vi "Reactivity Fitting.vi"() -> ()   [LabVIEW 2020]
uses:
  <vilib>/Utility/miscctls.llb/LVAnnotationListTypeDef.ctl
  global/SettingVariable.vi
  <vilib>/Analysis/NI_AALPro.lvlib
panel:
  out "反应性相对偏差":dbl[](array[numeric]) caption="相对偏差 (%)"
  out "最小二乘周期":dbl[](array[numeric]) caption="最小二乘法拟合 (s)"
  out "广义指数周期":dbl[](array[numeric]) caption="广义指数拟合 (s)"
  out "实测平均反应性":dbl[](array[numeric]) caption="实测平均值 (pcm)"
  out "周期法反应性":dbl[](array[numeric]) caption="周期法 (pcm)"
  out "采样间隔":dbl
  out "开始时间":timestamp
  in  "打开文件":bool
  out "历史波形图":cluster{dbl, dbl, dbl[][]}(graph)
  out "左选标时刻":timestamp caption="左选标时刻：" format="%<%.2X %x>T"
  out "数据点数":i32 caption="选中的数据点数："
  out "反应性记录表":string[][](table) caption="计算结果记录表"
  in  "保存表格":bool
  in  "添加记录":bool
  out "提示信息":string="打开文件后，拖动波形图中的游标选取临界段、动态段和终端段数据进行计算。"
  out "文件信息":string
  # "周期计算结果"
  # "反应性计算结果"
  # "坐标轴与图例"
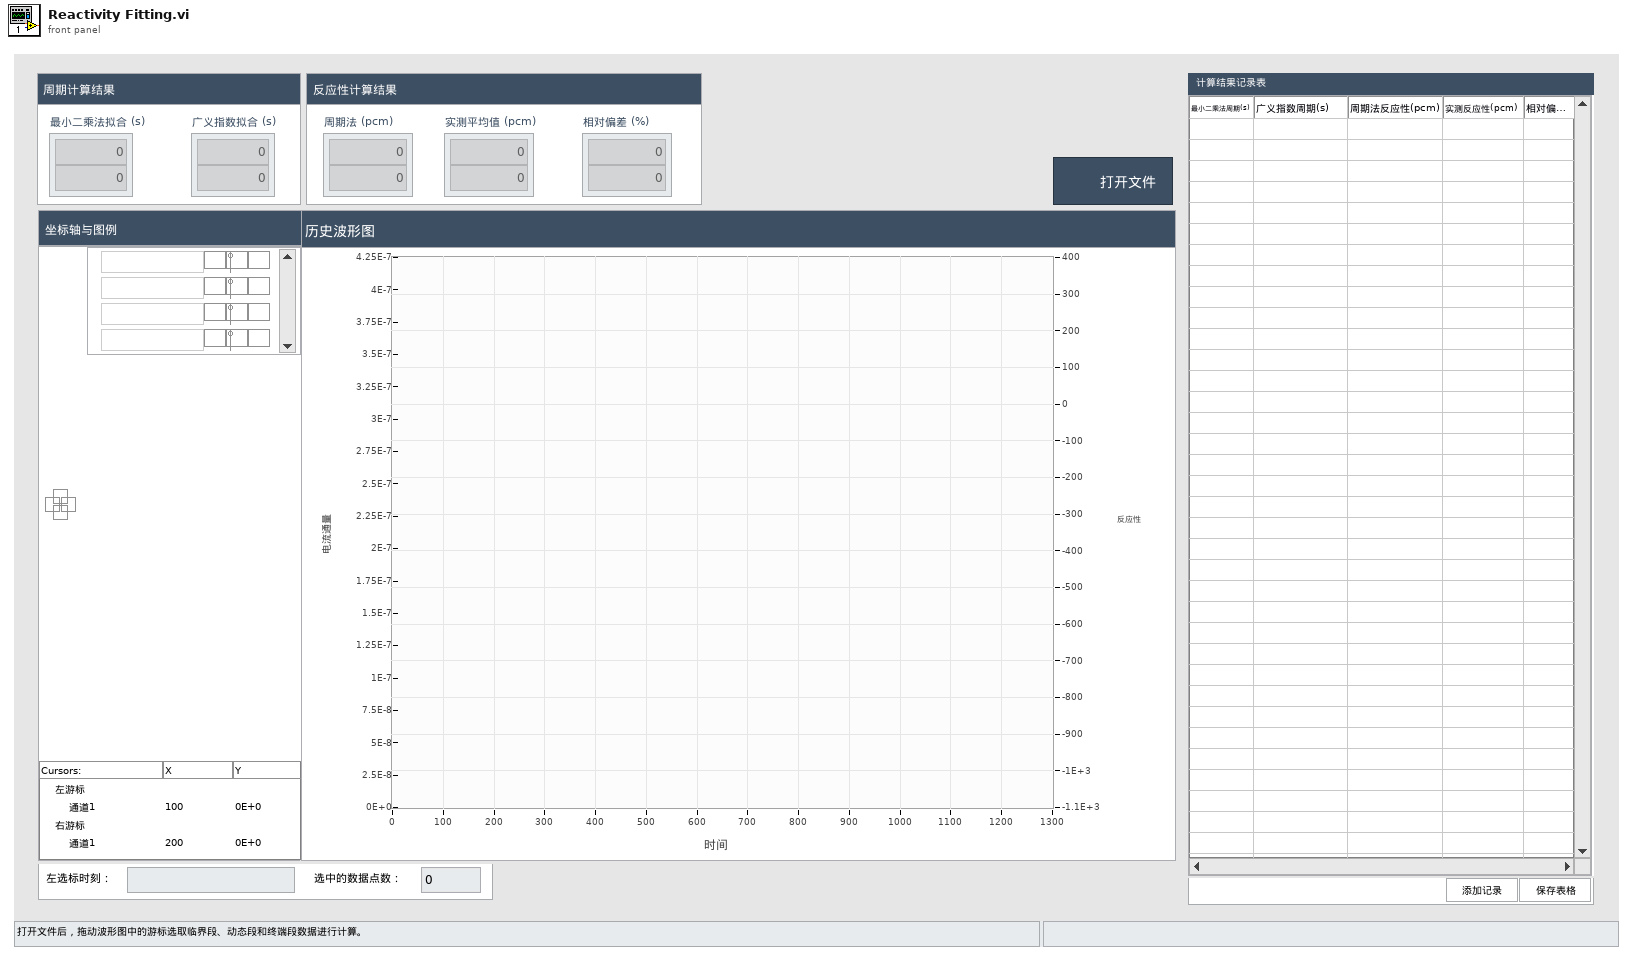
[diagram p1: front panel]
types:
  T1 = typedef "LVAnnotationListTypeDef.ctl" = cluster{"Name":string, "Color":u32, "Style":u8, "Point Style":u8, "Name Visible":bool, "Allow Drag":bool, "Annotation Mode":u32, "Plot":i32, "Index":i32, "Position":cluster{"X":dbl, "Y":dbl}, "X Scale":u32, "Y Scale":u32, "Show Arrow":bool, "Lock Name":bool, "Plot Area":i32, "Label Offset":cluster{"X":dbl, "Y":dbl}}[]
  T2 = cluster{"Name":string, "Color":u32, "Style":u8, "Point Style":u8, "Name Visible":bool, "Allow Drag":bool, "Annotation Mode":u32, "Plot":i32, "Index":i32, "Position":cluster{"X":dbl, "Y":dbl}, "X Scale":u32, "Y Scale":u32, "Show Arrow":bool, "Lock Name":bool, "Plot Area":i32, "Label Offset":cluster{"X":dbl, "Y":dbl}}
  T3 = cluster{"amp min":dbl, "amp max":dbl, "damping min":dbl, "damping max":dbl, "offset min":dbl, "offset max":dbl}
  T4 = enum16{"open", "replace", "create", "open or create", "replace or create", "replace or create with confirmation"}
  T5 = typedef "LVCursorListTypeDef.ctl" = cluster{"Name":string, "Color":u32, "Style":u8, "Point Style":u8, "Name Visible":bool, "Allow Drag":bool, "Cursor Mode":u32, "Plot":i32, "Index":i32, "Position":cluster{"X":dbl, "Y":dbl}, "X Scale":u32, "Y Scale":u32, "Watch Plots":i32[], "Watch All Plots":bool, "Plot Area":i32, "Label Offset":cluster{"X":dbl, "Y":dbl}}[]
  T6 = cluster{"Name":string, "Color":u32, "Style":u8, "Point Style":u8, "Name Visible":bool, "Allow Drag":bool, "Cursor Mode":u32, "Plot":i32, "Index":i32, "Position":cluster{"X":dbl, "Y":dbl}, "X Scale":u32, "Y Scale":u32, "Watch Plots":i32[], "Watch All Plots":bool, "Plot Area":i32, "Label Offset":cluster{"X":dbl, "Y":dbl}}
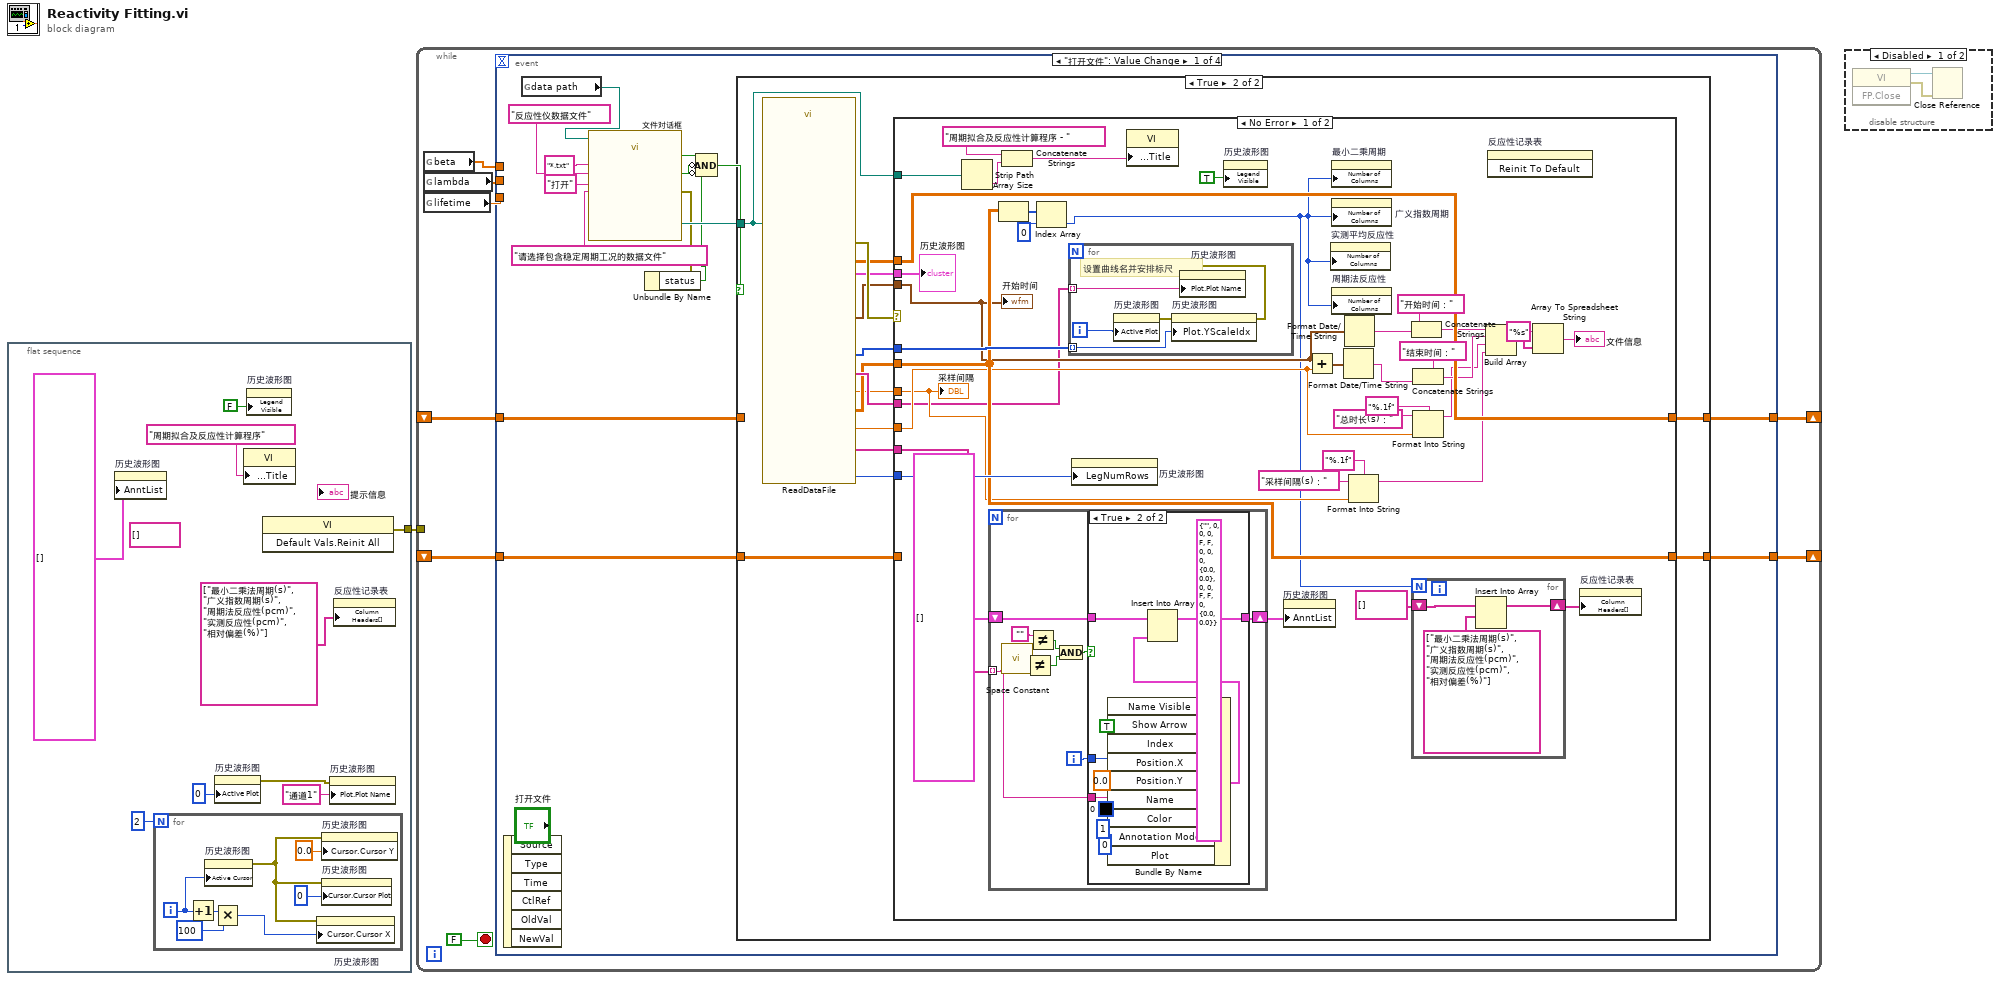
[diagram p0: block diagram]
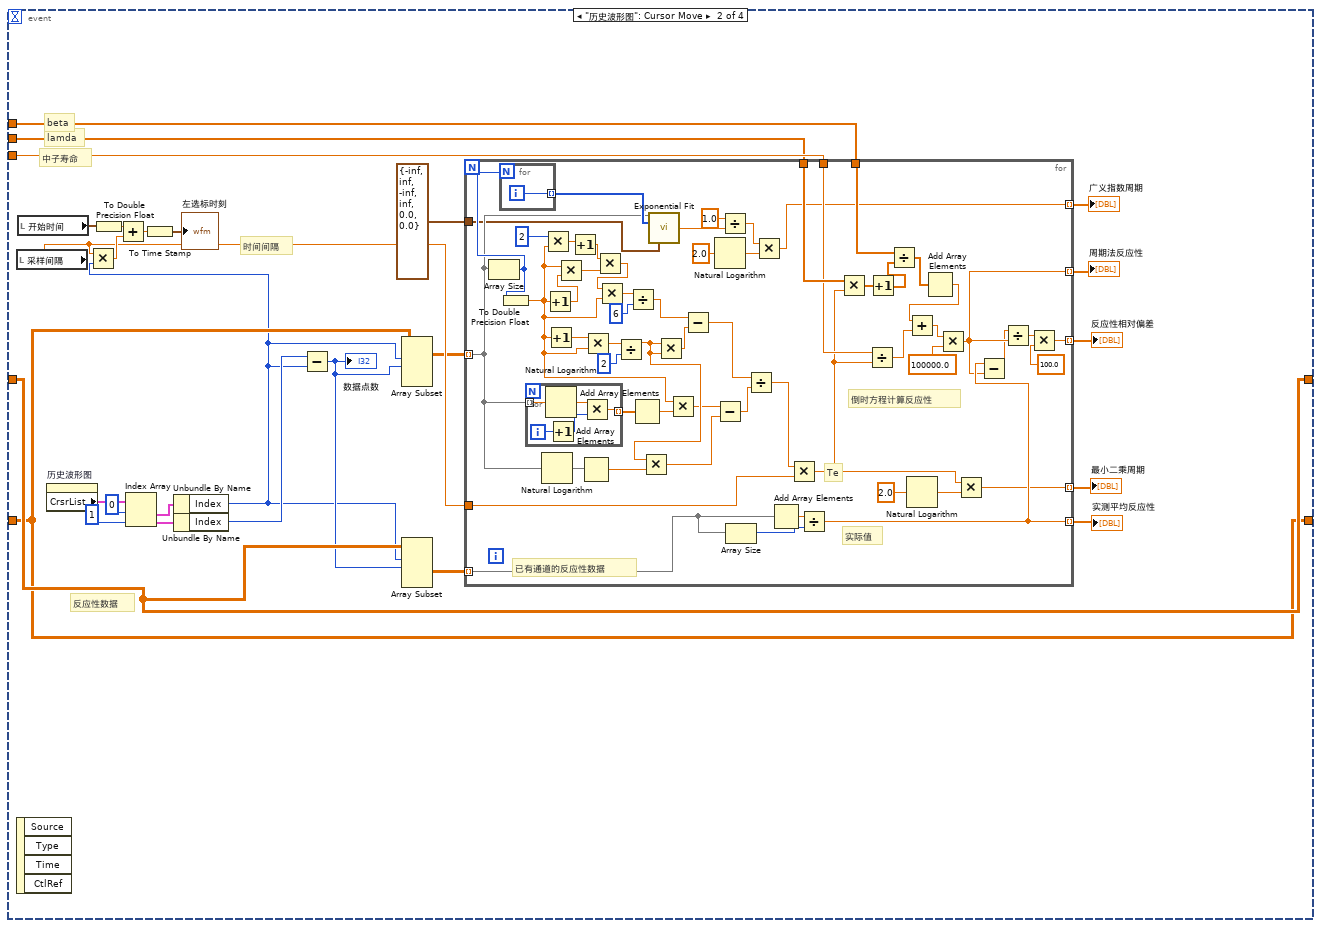
[diagram p5: hidden frame]
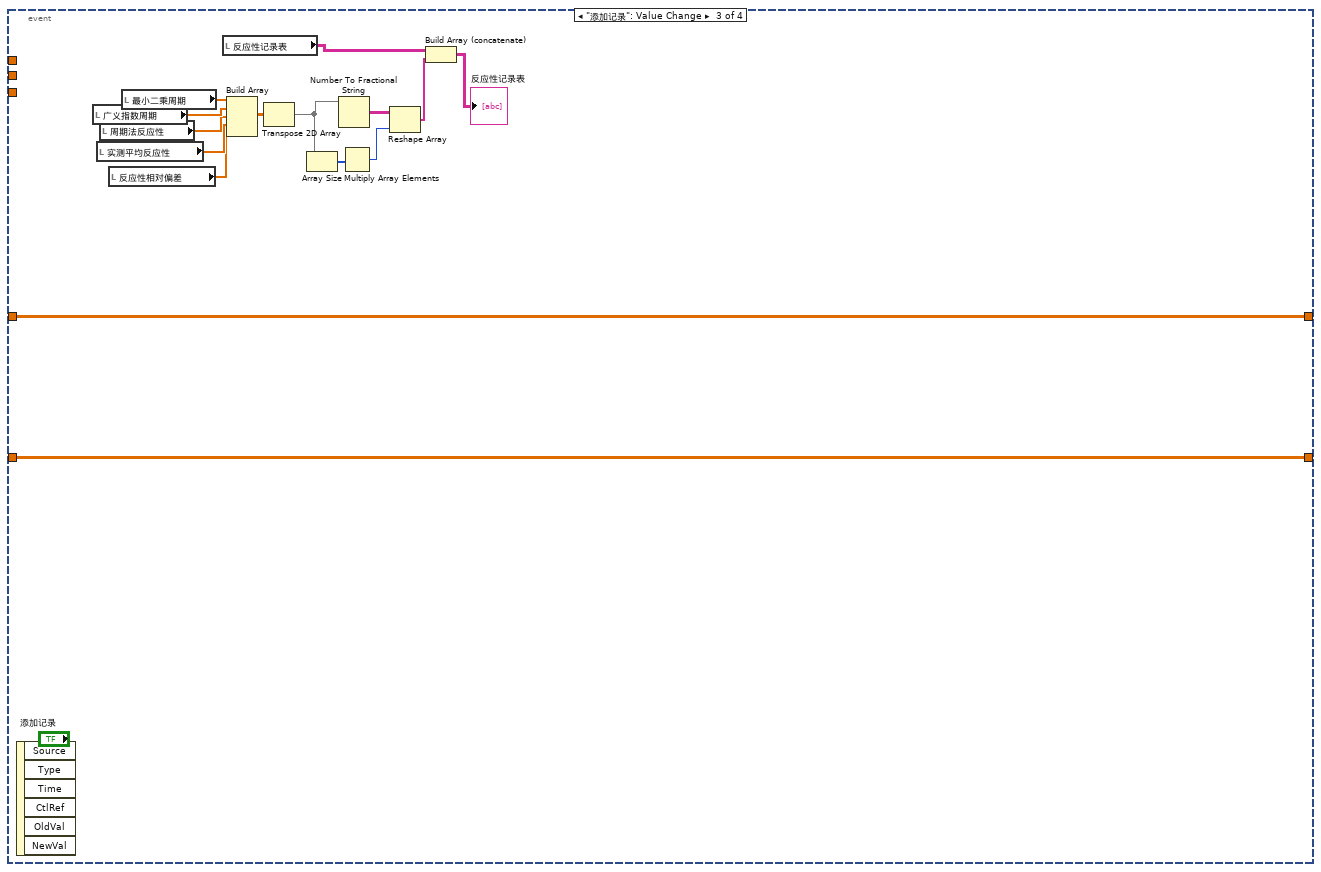
[diagram p6: hidden frame]
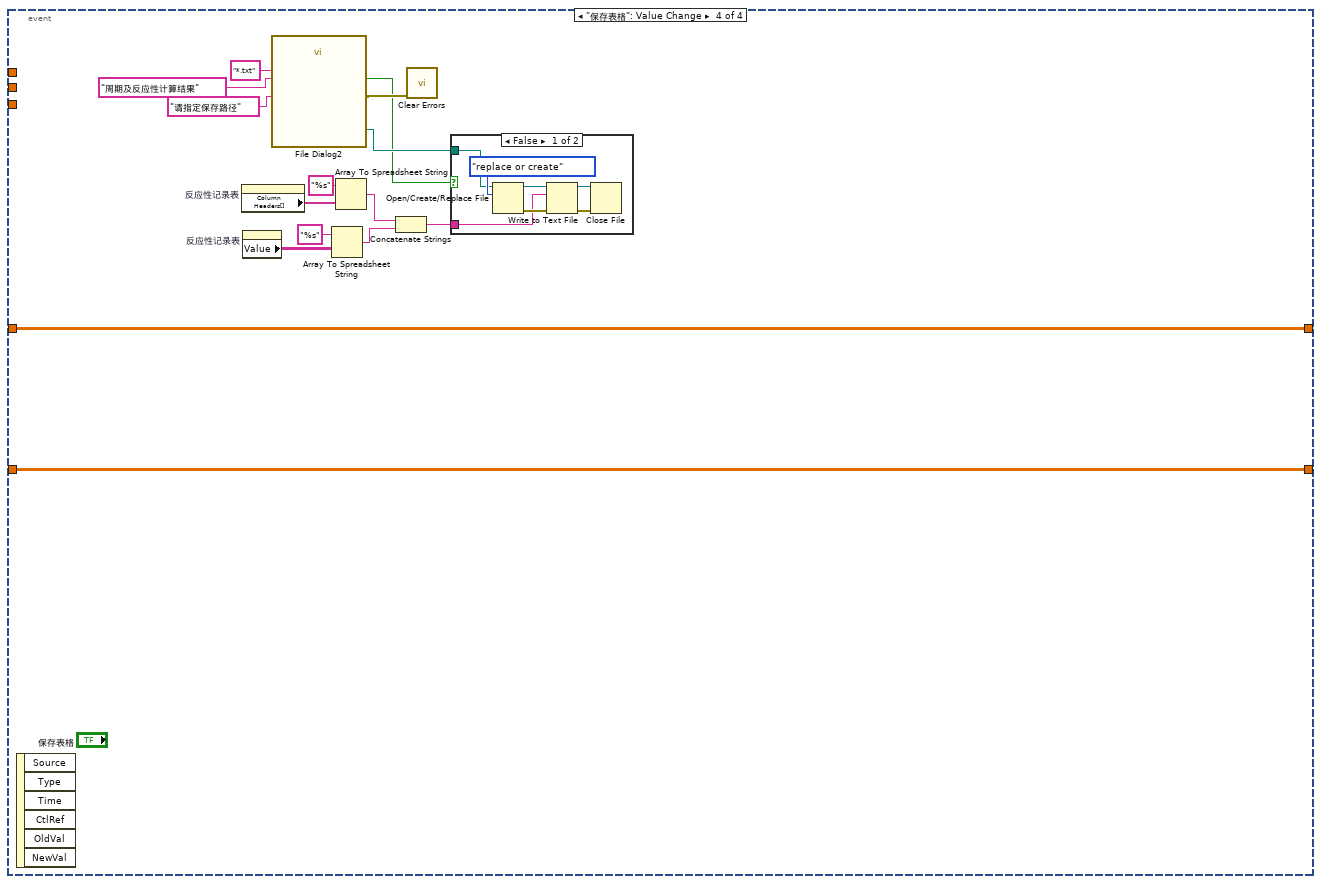
[diagram p7: hidden frame]
diagram:
  n1 = flat-sequence {
    tunnel: [w6] -> w1
    frame #0 {
      (unwired) string[] [] ("Strings []")
      n2 = property on="历史波形图" class="WFGraph (strict)"("AnntList"=T1 [] ("Annotation List")) -> ()  [unwired: 2 in, 2 out]
      n3 = for {
        N: 2 -> [_]
        i -> [w15]
        n4 = Increment(x=w15) -> (x+1=w14:i32)
        n5 = property on="历史波形图" class="WFGraph (strict)"("Active Cursor"=w15) -> (error out=w11:errorcluster)  [unwired: 2 in, 1 out]
        n6 = Multiply(x=w14, y=100) -> (x*y=w12:i32)
        n7 = property on="历史波形图" class="WFGraph (strict)"(error in=w11, "Cursor.Cursor X"=w12) -> ()  [unwired: 1 in, 2 out]
        n8 = property on="历史波形图" class="WFGraph (strict)"(error in=w11, "Cursor.Cursor Y"=0.0 ("Cursor.Cursor Position:Cursor Y")) -> ()  [unwired: 1 in, 2 out]
        n9 = property on="历史波形图" class="WFGraph (strict)"(error in=w11, "Cursor.Cursor Plot"=0 ("Cursor.Cursor Index")) -> ()  [unwired: 1 in, 2 out]
      }
      n10 = property on="历史波形图" class="WFGraph (strict)"("Active Plot"=u32 0) -> (error out=w8:errorcluster)  [unwired: 2 in, 1 out]
      n11 = property class="VI"("Front Panel.Title"="周期拟合及反应性计算程序" ("Front Panel Window:Title")) -> ()  [unwired: 2 in, 2 out]
      n12 = property on="历史波形图" class="WFGraph (strict)"("Legend Visible"=FALSE ("Legend:Visible")) -> ()  [unwired: 2 in, 2 out]
      n13 = invoke class="VI" method="Default Vals.Reinit All"() -> (error out=w6:errorcluster)  [unwired: 3 in, 2 out]
      n14 = property on="历史波形图" class="WFGraph (strict)"(error in=w8, "Plot.Plot Name"="通道1") -> ()  [unwired: 1 in, 2 out]
      n15 = property on="反应性记录表" class="Tbl (strict)"("Column Headers[]"=string[] ["最小二乘法周期(s)", "广义指数周期(s)", "周期法反应性(pcm)", "实测反应性(pcm)", "相对偏差(%)"] ("行首字符串[]")) -> ()  [unwired: 2 in, 2 out]
    }
  }
  n16 = while {
    shift-right: [w24] -> _
    shift-left: _ -> [w23]
    shift-right: [w22] -> _
    shift-left: _ -> [w21]
    tunnel: w1 -> [_]
    stop <- FALSE stop-if-true
    n17 = global read "SettingVariable.vi" "beta"() -> (w20:dbl[])
    n18 = global read "SettingVariable.vi" "lambda"() -> (w19:dbl[])
    n19 = global read "SettingVariable.vi" "lifetime"() -> (w18:dbl)
    n20 = event shown="[0] \"打开文件\": Value Change" {
      selector: _ -> [_ _ _ _]
      dyn-events: _ -> [_ _ _ _]
      timeout: _ -> [_ _ _ _]
      tunnel: [w35 w129 w231 w246] -> w24
      tunnel: w23 -> [w34 w129 w231 w246]
      tunnel: [w33 w143 w232 w247] -> w22
      tunnel: w21 -> [w32 w143 w232 w247]
      tunnel: w20 -> [_ w134 _ _]
      tunnel: w18 -> [_ w135 _ _]
      tunnel: w19 -> [_ w133 _ _]
      event "打开文件": Value Change {
        n21 = event-data() -> ()  [unwired: 1 in, 6 out]
        n22 = global read "SettingVariable.vi" "data path"() -> (w26:path)
        n23 = call "文件对话框"("start path"=w26, "prompt"="请选择包含稳定周期工况的数据文件", "button label"="打开", "pattern (all files)"="*.txt", "pattern label"="反应性仪数据文件") -> ("selected path"=w40:path, "exists"=w30:bool, "cancelled"=w29:bool, "error out"=w31:errorcluster)  [unwired: 7 in]
        n24 = Unbundle By Name(w31) -> ("status"=w28:bool)
        n25 = Compound Arithmetic op=AND(w30, invert w29, invert w28) -> (w27:bool)
        n26 = case shown="True" w27 {
          tunnel: w40 -> [_ w43]
          tunnel: [w42 w49] -> w35
          tunnel: w34 -> [w42 w48]
          tunnel: [w41 w45] -> w33
          tunnel: w32 -> [w41 _]
          frame False {
          }
          frame True {
            n27 = call "ReadDataFile.vi"("file path (dialog if empty)"=w43) -> ("曲线对应标尺编号"=w52:i32[], "曲线名"=w51:string[], "通量数据"=w50:dbl[][], "时间间隔"=w47:dbl, "曲线数"=w54:i32, "开始时间"=w44:timestamp, "反应性数据"=w46:dbl[][], "总时长(s)"=w55:dbl, "error out"=w57:errorcluster, "备注数组"=w53:string[], "波形簇"=w56:cluster{dbl, dbl, dbl[][]})  [unwired: 2 in, 2 out]
            n28 = case shown="No Error" w57 {
              tunnel: w56 -> [w95 _]
              tunnel: w55 -> [w77 _]
              tunnel: w54 -> [w94 _]
              tunnel: w53 -> [w91 _]
              tunnel: w52 -> [w90 _]
              tunnel: w51 -> [w64 _]
              tunnel: w50 -> [w87 _]
              tunnel: [w87 w126] -> w49
              tunnel: w48 -> [_ w126]
              tunnel: w47 -> [w75 _]
              tunnel: w46 -> [w86 w125]
              tunnel: [w86 w125] -> w45
              tunnel: w44 -> [w82 _]
              tunnel: w43 -> [w59 _]
              frame No Error {
                n29 = Strip Path(path=w59) -> (name=w60:string)  [unwired: 1 out]
                n30 = for {
                  tunnel: w91 -> [w107] mode=indexing
                  shift-right: [w109] -> w93
                  shift-left: T1 [] ("注释列表") -> [w110]
                  i -> [w111]
                  n31 = call <vilib>:"Space Constant.vi"() -> ("String"=w112:string)
                  n32 = Not Equal?(x=w112, y=w107) -> (x != y?=w105:bool)
                  n33 = Not Equal?(x="", y=w107) -> (x != y?=w106:bool)
                  n34 = And(x=w106, y=w105) -> (x .and. y?=w104:bool)
                  n35 = case shown="True" w104 {
                    tunnel: w107 -> [_ w119]
                    tunnel: w111 -> [_ w121]
                    tunnel: w110 -> [w113 w124]
                    tunnel: [w113 w123] -> w109
                    frame False {
                    }
                    frame True {
                      w122 = TRUE ("Show Arrow")
                      n36 = Bundle By Name(cluster=T2 {"Name"="", "Color"=0, "Style"=0, "Point Style"=0, "Name Visible"=FALSE, "Allow Drag"=FALSE, "Annotation Mode"=0, "Plot"=0, "Index"=0, "Position"={"X"=0.0, "Y"=0.0}, "X Scale"=0, "Y Scale"=0, "Show Arrow"=FALSE, "Lock Name"=FALSE, "Plot Area"=0, "Label Offset"={"X"=0.0, "Y"=0.0}} ("元素"), "Name Visible"=w122, "Show Arrow"=w122, "Index"=w121, "Position.X"=w121, "Position.Y"=0.0 ("Y"), "Name"=w119, "Color"=u32 0, "Annotation Mode"=u32 1, "Plot"=0) -> (w120:T2)
                      n37 = Insert Into Array(array=w124, new element=w120) -> (w123:T1)  [unwired: 1 in]
                    }
                  }
                }
                n38 = Array Size(array=w87) -> (size(s)=w89:i32[])
                n39 = Concatenate Strings("周期拟合及反应性计算程序 - " ("string"), w60) -> (w61:string)
                n40 = Index Array(array=w89, index=0 ("索引")) -> (element=w63:i32)
                n41 = for {
                  tunnel: w90 -> [w101] mode=indexing
                  tunnel: w64 -> [w99] mode=indexing
                  i -> [w100]
                  # "设置曲线名并安排标尺"
                  n42 = property on="历史波形图" class="WFGraph (strict)"("Active Plot"=w100) -> (error out=w103:errorcluster)  [unwired: 2 in, 1 out]
                  n43 = property on="历史波形图" class="WFGraph (strict)"(error in=w103, "Plot.YScaleIdx"=w101) -> (error out=w102:errorcluster)  [unwired: 1 in, 1 out]
                  n44 = property on="历史波形图" class="WFGraph (strict)"(error in=w102, "Plot.Plot Name"=w99) -> ()  [unwired: 1 in, 2 out]
                }
                n45 = property on="历史波形图" class="WFGraph (strict)"("LegNumRows"=w94) -> ()  [unwired: 2 in, 2 out]
                n46 = property class="VI"("Front Panel.Title"=w61) -> ()  [unwired: 2 in, 2 out]
                n47 = property on="历史波形图" class="WFGraph (strict)"("Legend Visible"=TRUE ("Legend:Visible")) -> ()  [unwired: 2 in, 2 out]
                n48 = property on="历史波形图" class="WFGraph (strict)"("AnntList"=w93) -> ()  [unwired: 2 in, 2 out]
                n49 = Add(x=w82, y=w77) -> (x+y=w83:timestamp)
                n50 = property on="实测平均反应性" class="Arr (strict)"("Number of Columns"=w63) -> ()  [unwired: 2 in, 2 out]
                n51 = property on="最小二乘周期" class="Arr (strict)"("Number of Columns"=w63) -> ()  [unwired: 2 in, 2 out]
                n52 = property on="广义指数周期" class="Arr (strict)"("Number of Columns"=w63) -> ()  [unwired: 2 in, 2 out]
                n53 = property on="周期法反应性" class="Arr (strict)"("Number of Columns"=w63) -> ()  [unwired: 2 in, 2 out]
                n54 = Format Date/Time String(seconds (now)=w83) -> (date/time string=w78:string)  [unwired: 2 in]
                n55 = Format Date/Time String(seconds (now)=w82) -> (date/time string=w80:string)  [unwired: 2 in]
                n56 = Format Into String(format string="%.1f", initial string="采样间隔(s)：", w75) -> (resulting string=w68:string)  [unwired: 1 in, 1 out]
                n57 = Concatenate Strings("开始时间：" ("string"), w80) -> (w73:string)
                n58 = for {
                  N: w63 -> [_]
                  shift-right: [w96] -> w84
                  shift-left: string[] [] ("行首字符串[]") -> [w97]
                  n59 = Insert Into Array(array=w97, new element=string[] ["最小二乘法周期(s)", "广义指数周期(s)", "周期法反应性(pcm)", "实测反应性(pcm)", "相对偏差(%)"] ("行首字符串[]")) -> (w96:string[])  [unwired: 1 in]
                }
                n60 = Concatenate Strings("结束时间：" ("string"), w78) -> (w70:string)
                n61 = Format Into String(format string="%.1f", initial string="总时长(s)：", w77) -> (resulting string=w69:string)  [unwired: 1 in, 1 out]
                n62 = Build Array(w73, w70, w69, w68) -> (w72:string[])
                n63 = invoke on="反应性记录表" class="Tbl (strict)" method="Reinit To Default"() -> ()  [unwired: 3 in, 3 out]
                n64 = Array To Spreadsheet String(array=w72, 3:"%s" ("format string")) -> (spreadsheet string=→"文件信息":string)  [unwired: 1 in]
                n65 = property on="反应性记录表" class="Tbl (strict)"("Column Headers[]"=w84) -> ()  [unwired: 2 in, 2 out]
                "历史波形图" <- w95
                "开始时间" <- w82
                "采样间隔" <- w75
              }
              frame Error {
              }
            }
          }
        }
      }
      event "历史波形图": Cursor Move {
        # "lamda"
        # "beta"
        # "中子寿命"
        # "反应性数据"
        # "时间间隔"
        n66 = local read "采样间隔"() -> (w132:dbl)
        n67 = event-data() -> ()  [unwired: 1 in, 4 out]
        n68 = local read "开始时间"() -> (w142:timestamp)
        n69 = property on="历史波形图" class="WFGraph (strict)"() -> ("CrsrList"=w149:T5)  [unwired: 2 in, 2 out]
        n70 = To Double Precision Float(number=w142) -> (double precision float=w148:dbl)
        n71 = Index Array(array=w149, index #1=0 ("index"), index #2=1 ("index")) -> (element #1=w151:T6, element #2=w153:T6)
        n72 = Unbundle By Name(w151) -> ("Index"=w127:i32)
        n73 = Multiply(x=w132, y=w127) -> (x*y=w145:dbl)
        n74 = Add(x=w148, y=w145) -> (x+y=w147:dbl)
        n75 = To Time Stamp(1:w147) -> (0:→"左选标时刻":timestamp)
        n76 = Unbundle By Name(w153) -> ("Index"=w144:i32)
        n77 = Subtract(x=w144, y=w127) -> (x-y=w128:i32)
        "数据点数" <- w128
        n78 = Array Subset(array=w129, index (row)=w127, length (row)=w128) -> (w130:dbl[][])  [unwired: 2 in]
        n79 = Array Subset(array=w143, index (row)=w127, length (row)=w128) -> (w131:dbl[][])  [unwired: 2 in]
        n80 = for {
          tunnel: w130 -> [w162] mode=indexing
          tunnel: w135 -> [w205]
          tunnel: w134 -> [w211]
          tunnel: w133 -> [w210]
          tunnel: w131 -> [w203] mode=indexing
          tunnel: [w209] -> w139 mode=indexing
          tunnel: [w208] -> w137 mode=indexing
          tunnel: [w207] -> w136 mode=indexing
          tunnel: [w204] -> w138 mode=indexing
          tunnel: w132 -> [w206]
          tunnel: [w155] -> w140 mode=indexing
          tunnel: T3 {"amp min"=-inf, "amp max"=inf, "damping min"=-inf, "damping max"=inf, "offset min"=0.0, "offset max"=0.0} ("parameter bounds") -> [w154]
          # "已有通道的反应性数据"
          # "倒时方程计算反应性"
          # "实际值"
          # "Te"
          n81 = Array Size(array=w162) -> (size(s)=w164:i32)
          n82 = for {
            N: w164 -> [_]
            tunnel: [w212] -> w163 mode=indexing
            i -> [w212]
          }
          n83 = To Double Precision Float(number=w164) -> (double precision float=w168:dbl)
          n84 = for {
            tunnel: w162 -> [w217] mode=indexing
            tunnel: [w213] -> w180 mode=indexing
            i -> [w216]
            n85 = Natural Logarithm(1:w217) -> (0:w215:dbl)
            n86 = Increment(x=w216) -> (x+1=w214:i32)
            n87 = Multiply(x=w215, y=w214) -> (x*y=w213:dbl)
          }
          n88 = Natural Logarithm(1:w162) -> (0:w175:dbl[])
          n89 = Multiply(x=2 ("count"), y=w168) -> (x*y=w187:dbl)
          n90 = Increment(x=w168) -> (x+1=w190:dbl)
          n91 = Increment(x=w168) -> (x+1=w184:dbl)
          n92 = Multiply(x=w168, y=w190) -> (x*y=w188:dbl)
          n93 = Increment(x=w187) -> (x+1=w186:dbl)
          n94 = Add Array Elements(numeric array=w175) -> (sum=w174:dbl)
          n95 = Multiply(x=w184, y=w168) -> (x*y=w183:dbl)
          n96 = Multiply(x=w186, y=w188) -> (x*y=w185:dbl)
          n97 = Multiply(x=w185, y=w168) -> (x*y=w171:dbl)
          n98 = Divide(x=w183, y=2 ("count")) -> (x/y=w178:dbl)
          n99 = Divide(x=w171, y=6 ("count")) -> (x/y=w169:dbl)
          n100 = Add Array Elements(numeric array=w180) -> (sum=w181:dbl)
          n101 = Multiply(x=w178, y=w174) -> (x*y=w176:dbl)
          n102 = call <vilib>:"Exponential Fit.vi"("Y"=w162, "X"=w163, "parameter bounds"=w154) -> ("damping"=w160:dbl)  [unwired: 7 in, 5 out]
          n103 = Multiply(x=w178, y=w178) -> (x*y=w179:dbl)
          n104 = Multiply(x=w168, y=w181) -> (x*y=w177:dbl)
          n105 = Subtract(x=w169, y=w179) -> (x-y=w172:dbl)
          n106 = Natural Logarithm(1:sgl 2.0) -> (0:w156:sgl)
          n107 = Subtract(x=w177, y=w176) -> (x-y=w173:dbl)
          n108 = Divide(x=1.0, y=w160) -> (x/y=w157:dbl)
          n109 = Array Size(array=w203) -> (size(s)=w191:i32)
          n110 = Divide(x=w172, y=w173) -> (x/y=w161:dbl)
          n111 = Multiply(x=w157, y=w156) -> (x*y=w155:dbl)
          n112 = Add Array Elements(numeric array=w203) -> (sum=w202:dbl)
          n113 = Multiply(x=w161, y=w206) -> (x*y=w165:dbl)
          n114 = Divide(x=w202, y=w191) -> (x/y=w208:dbl)
          n115 = Multiply(x=w210, y=w165) -> (x*y=w192:dbl[])
          n116 = Divide(x=w205, y=w165) -> (x/y=w199:dbl)
          n117 = Increment(x=w192) -> (x+1=w193:dbl[])
          n118 = Divide(x=w211, y=w193) -> (x/y=w201:dbl[])
          n119 = Natural Logarithm(1:sgl 2.0) -> (0:w167:sgl)
          n120 = Add Array Elements(numeric array=w201) -> (sum=w200:dbl)
          n121 = Add(x=w200, y=w199) -> (x+y=w198:dbl)
          n122 = Multiply(x=w198, y=sgl 100000.0) -> (x*y=w207:dbl)
          n123 = Multiply(x=w165, y=w167) -> (x*y=w204:dbl)
          n124 = Subtract(x=w208, y=w207) -> (x-y=w197:dbl)
          n125 = Divide(x=w197, y=w207) -> (x/y=w196:dbl)
          n126 = Multiply(x=w196, y=sgl 100.0) -> (x*y=w209:dbl)
        }
        "周期法反应性" <- w136
        "实测平均反应性" <- w137
        "广义指数周期" <- w140
        "最小二乘周期" <- w138
        "反应性相对偏差" <- w139
      }
      event "添加记录": Value Change {
        n127 = event-data() -> ()  [unwired: 1 in, 6 out]
        n128 = local read "广义指数周期"() -> (w229:dbl[])
        n129 = local read "实测平均反应性"() -> (w227:dbl[])
        n130 = local read "周期法反应性"() -> (w228:dbl[])
        n131 = local read "反应性相对偏差"() -> (w218:dbl[])
        n132 = local read "最小二乘周期"() -> (w230:dbl[])
        n133 = local read "反应性记录表"() -> (w225:string[][])
        n134 = Build Array(w230, w229, w228, w227, w218) -> (w219:dbl[][])
        n135 = Transpose 2D Array(2D array=w219) -> (transposed array=w220:dbl[][])
        n136 = Array Size(array=w220) -> (size(s)=w222:i32[])
        n137 = Number To Fractional String(number=w220) -> (F-format string=w226:string[][])  [unwired: 3 in]
        n138 = Multiply Array Elements(1:w222) -> (0:w221:i32)
        n139 = Reshape Array(w226, w221) -> (w224:string[])
        n140 = Build Array (concatenate)(w225, w224) -> (→"反应性记录表":string[][])
      }
      event "保存表格": Value Change {
        n141 = event-data() -> ()  [unwired: 1 in, 6 out]
        n142 = property on="反应性记录表" class="Tbl (strict)"() -> ("Column Headers[]"=w245:string[])  [unwired: 2 in, 2 out]
        n143 = property on="反应性记录表" class="Tbl (strict)"() -> ("Value"=w242:string[][])  [unwired: 2 in, 2 out]
        n144 = call "File Dialog2"("prompt"="请指定保存路径" ("提示"), "pattern (all files)"="*.txt" ("类型（所有文件）"), "pattern label"="周期及反应性计算结果" ("默认名称")) -> ("selected path"=w239:path, "cancelled"=w238:bool, "error out"=w240:errorcluster)  [unwired: 9 in, 1 out]
        n145 = Array To Spreadsheet String(array=w242, 3:"%s" ("format string")) -> (spreadsheet string=w241:string)  [unwired: 1 in]
        n146 = Array To Spreadsheet String(array=w245, 3:"%s" ("格式字符串")) -> (spreadsheet string=w244:string)  [unwired: 1 in]
        n147 = Concatenate Strings(w244, w241) -> (w243:string)
        n148 = call <vilib>:"Clear Errors.vi"("error in (no error)"=w240) -> ()  [unwired: 5 in, 2 out]
        n149 = case shown="False" w238 {
          tunnel: w243 -> [w249 _]
          tunnel: w239 -> [w248 _]
          frame False {
            n150 = Open/Create/Replace File(file path (use dialog)=w248, operation (0:open)=T4."replace or create") -> (refnum out=w252:refnum<file>, error out=w254:errorcluster)  [unwired: 4 in, 1 out]
            n151 = Write to Text File(file (use dialog)=w252, text=w249, error in=w254) -> (refnum out=w251:refnum<file>, error out=w250:errorcluster)  [unwired: 1 in, 1 out]
            n152 = Close File(refnum=w251, error in=w250) -> ()  [unwired: 2 out]
          }
          frame True {
          }
        }
      }
    }
  }
  n153 = disable-structure shown="Disabled" {
    frame Disabled {
      n154 = invoke class="VI" method="FP.Close"() -> (reference out=w256:refnum<vi>, error out=w255:errorcluster)  [unwired: 3 in, 1 out]
      n155 = Close Reference(reference=w256, error in (no error)=w255) -> ()  [unwired: 1 out]
    }
    frame Enabled {
    }
  }
